vi "Clear Faults Test.vi"() -> ()   [LabVIEW 2014]
uses:
  Controls/Gen Data.ctl
  Controls/ES System Data.ctl
  Controls/StringSelector.ctl
  Controls/PC Data.ctl
  Controls/MicroZed Config Op Mode.ctl
  Controls/FPGA Data.ctl
panel:
  out "Startup":bool
  out "Wait for Fault":bool
  in  "Shutdown?":bool
  out "Error Out":errorcluster
  out "Clear Error":bool
  out "Manual Shutdown":bool
  in  "Error In":errorcluster
  in  "FPGA Data":T1 {"SSG Active Current" format="%2.1f"; "PV Reactive Power (L1)" format="%2.1f"; "PV Reactive Power (L2)" format="%2.1f"; "PV Total Reactive Power" format="%2.1f"; "Gen Reactive Power (L1)" format="%2.1f"; "Gen Reactive Power (L2)" format="%2.1f"; "Gen Total Reactive Power" format="%2.1f"; "SSG Reactive Power (L1)" format="%2.1f"; "SSG Reactive Power (L2)" format="%2.1f"; "SSG Total Reactive Power" format="%2.1f"; "PV Total Current" format="%2.1f"; "PV Total Voltage" format="%2.1f"; "PV Active Power (L1)" format="%2.1f"; "PV Active Power (L2)" format="%2.1f"; "PV App Power (L1)" format="%2.1f"; "PV App Power (L2)" format="%2.1f"; "PV Total Active Power" format="%2.1f"; "PV Total App Power" format="%2.1f"; "PV Arms (L1)" format="%2.1f"; "PV Arms (L2)" format="%2.1f"; "PV Vrms (L1)" format="%2.1f"; "PV Vrms (L2)" format="%2.1f"; "Gen Total Current" format="%2.1f"; "SSG Total Current" format="%2.1f"; "Gen Total Voltage" format="%2.1f"; "SSG Total Voltage" format="%2.1f"; "Gen Active Power (L1)" format="%2.1f"; "Gen Active Power (L2)" format="%2.1f"; "SSG Active Power (L1)" format="%2.1f"; "SSG Active Power (L2)" format="%2.1f"; "Gen App Power (L1)" format="%2.1f"; "Gen App Power (L2)" format="%2.1f"; "SSG App Power (L1)" format="%2.1f"; "SSG App Power (L2)" format="%2.1f"; "Gen Total Active Power" format="%2.1f"; "Gen Total App Power" format="%2.1f"; "Gen Arms (L1)" format="%2.1f"; "Gen Arms (L2)" format="%2.1f"; "Gen Vrms (L1)" format="%2.1f"; "Gen Vrms (L2)" format="%2.1f"; "SSG Total Active Power" format="%2.1f"; "SSG Total App Power" format="%2.1f"; "SSG Arms (L1)" format="%2.1f"; "SSG Arms (L2)" format="%2.1f"; "SSG Vrms (L1)" format="%2.1f"; "SSG Vrms (L2)" format="%2.1f"}
  in  "PC Data":T2 {"Alarms 2" format="%016b"; "Faults 2" format="%016b"; "Alarms 1" format="%016b"; "Faults 1" format="%016b"; "Contactor FB" format="%.0b"; "DC Voltage SP" format="%2.1f"; "Clear Faults SP" format="%.0b"; "Neutral Current" format="%2.1f"; "AC Current - L2" format="%2.1f"; "AC Voltage - L2" format="%2.1f"; "Temperature" format="%2.1f"; "DC Voltage" format="%2.1f"; "AC Current SP" format="%2.1f"; "AC Voltage SP" format="%2.1f"; "Frequency SP" format="%2.1f"; "AC Frequency" format="%2.1f"; "AC Current - L1" format="%2.1f"; "AC Voltage- L1" format="%2.1f"}
  in  "ES System Data":T4={"Voltage"=0.0, "Current"=0.0, "SOC Avg"=0.0, "Faults"=0, "Alarms"=0, "# Strings"=0, "Max Temp"=0, "Min Temp"=0, "Max Cell Voltage"=0.0, "Min Cell Voltage"=0.0, "Energy Capacity"=0.0, "Energy Remaining"=0.0, "SOC Min"=0.0, "SOC Max"=0.0, "ES Fault"=FALSE, "String Select"=enum."3 Strings", "ES Com Fault"=FALSE, "SOH Avg"=0.0}
  in  "Gen Active":T6 {"Alarms" format="%04x"}
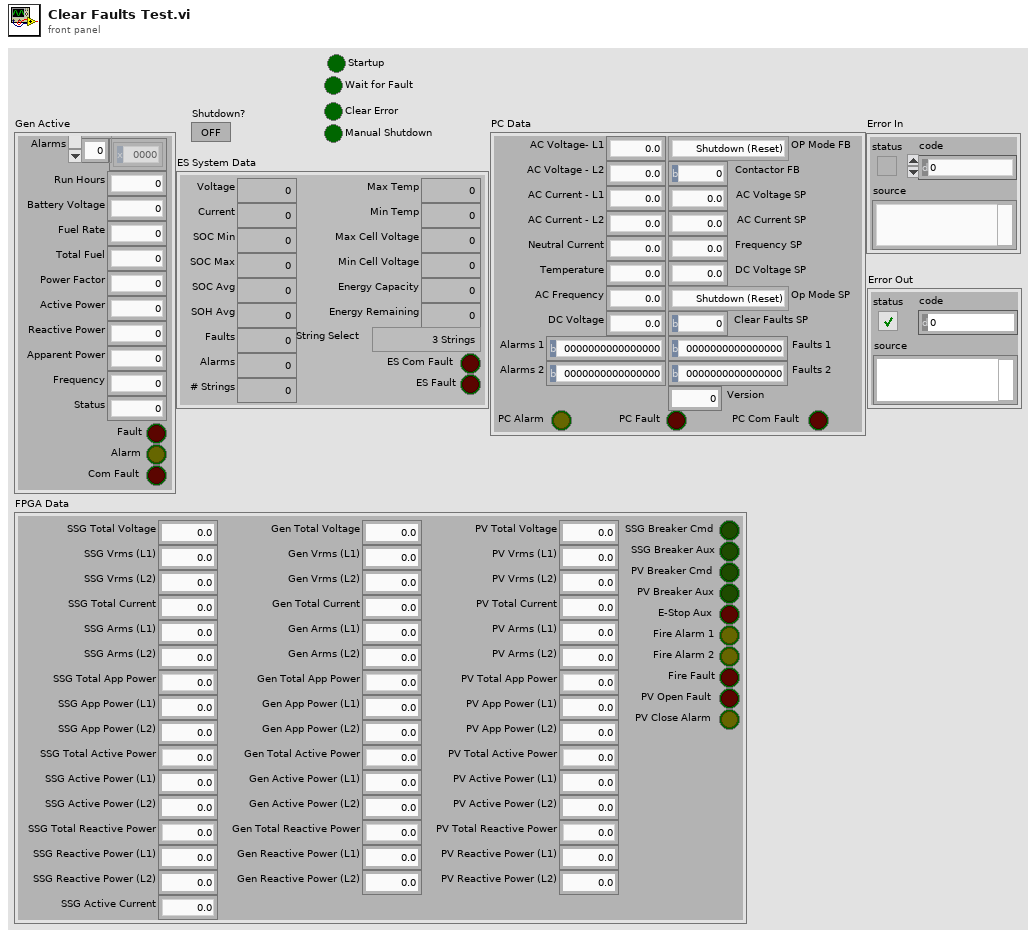
[diagram p1: front panel]
types:
  T1 = typedef "FPGA Data.ctl" = cluster{"Gen Total Voltage":dbl, "Gen Vrms (L1)":dbl, "Gen Vrms (L2)":dbl, "Gen Total Current":dbl, "Gen Arms (L1)":dbl, "Gen Arms (L2)":dbl, "Gen Total App Power":dbl, "Gen App Power (L1)":dbl, "Gen App Power (L2)":dbl, "Gen Total Active Power":dbl, "Gen Active Power (L1)":dbl, "Gen Active Power (L2)":dbl, "Gen Total Reactive Power":dbl, "Gen Reactive Power (L1)":dbl, "Gen Reactive Power (L2)":dbl, "SSG Total Voltage":dbl, "SSG Vrms (L1)":dbl, "SSG Vrms (L2)":dbl, "SSG Total Current":dbl, "SSG Arms (L1)":dbl, "SSG Arms (L2)":dbl, "SSG Total App Power":dbl, "SSG App Power (L1)":dbl, "SSG App Power (L2)":dbl, "SSG Total Active Power":dbl, "SSG Active Power (L1)":dbl, "SSG Active Power (L2)":dbl, "SSG Total Reactive Power":dbl, "SSG Reactive Power (L1)":dbl, "SSG Reactive Power (L2)":dbl, "PV Total Voltage":dbl, "PV Vrms (L1)":dbl, "PV Vrms (L2)":dbl, "PV Total Current":dbl, "PV Arms (L1)":dbl, "PV Arms (L2)":dbl, "PV Total App Power":dbl, "PV App Power (L1)":dbl, "PV App Power (L2)":dbl, "PV Total Active Power":dbl, "PV Active Power (L1)":dbl, "PV Active Power (L2)":dbl, "PV Total Reactive Power":dbl, "PV Reactive Power (L1)":dbl, "PV Reactive Power (L2)":dbl, "SSG Breaker Cmd":bool, "SSG Breaker Aux":bool, "PV Breaker Cmd":bool, "PV Breaker Aux":bool, "E-Stop Aux":bool, "Fire Alarm 1":bool, "Fire Alarm 2":bool, "Fire Fault":bool, "PV Open Fault":bool, "PV Close Alarm":bool, "SSG Active Current":dbl}
  T2 = typedef "PC Data.ctl" = cluster{"AC Voltage- L1":dbl, "AC Voltage - L2":dbl, "AC Current - L1":dbl, "AC Current - L2":dbl, "Neutral Current":dbl, "Temperature":dbl, "AC Frequency":dbl, "DC Voltage":dbl, "AC Voltage SP":dbl, "AC Current SP":dbl, "Frequency SP":dbl, "Op Mode SP":T3, "Clear Faults SP":u16, "PC Com Fault":bool, "PC Fault":bool, "DC Voltage SP":dbl, "OP Mode FB":T3, "Contactor FB":u16, "Faults 1":u16, "Alarms 1":u16, "Faults 2":u16, "Alarms 2":u16, "PC Alarm":bool, "Version":u16}
  T3 = typedef "MicroZed Config Op Mode.ctl" = enum16{"Shutdown (Reset)", "Startup", "Idle", "Voltage Mode", "Current Mode", "Fault", "OL Voltage (Debug)", "No Data"}
  T4 = typedef "ES System Data.ctl" = cluster{"Voltage":sgl, "Current":sgl, "SOC Avg":sgl, "Faults":u16, "Alarms":u16, "# Strings":u16, "Max Temp":i16, "Min Temp":i16, "Max Cell Voltage":sgl, "Min Cell Voltage":sgl, "Energy Capacity":sgl, "Energy Remaining":sgl, "SOC Min":sgl, "SOC Max":sgl, "ES Fault":bool, "String Select":T5, "ES Com Fault":bool, "SOH Avg":sgl}
  T5 = typedef "StringSelector.ctl" = enum16{"1 String (1)", "1 String (2)", "1 String (3)", "2 Strings (1 2)", "2 Strings (2 3)", "2 Strings (1 3)", "3 Strings"}
  T6 = typedef "Gen Data.ctl" = cluster{"Alarms":i16[], "Run Hours":dbl, "Battery Voltage":dbl, "Fuel Rate":dbl, "Total Fuel":dbl, "Power Factor":dbl, "Active Power":dbl, "Reactive Power":dbl, "Apparent Power":dbl, "Frequency":dbl, "Status":u16, "Fault":bool, "Alarm":bool, "Com Fault":bool}
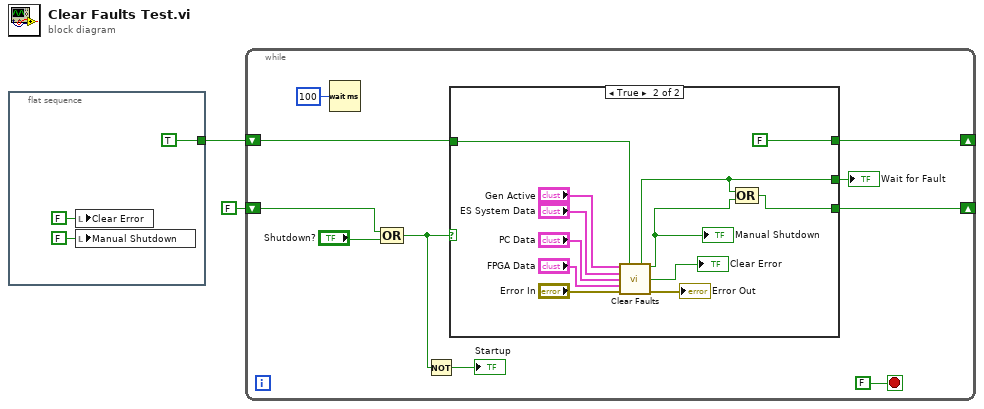
[diagram p0: block diagram]
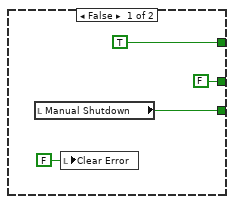
[diagram p2: hidden frame]
diagram:
  n1 = flat-sequence {
    tunnel: [TRUE] -> w2
    frame #0 {
      n2 = local write "Clear Error"(FALSE ("Clear Error")) -> ()
      n3 = local write "Manual Shutdown"(FALSE ("Manual Shutdown")) -> ()
    }
  }
  n4 = while {
    shift-right: [w12] -> _
    shift-left: w2 -> [w13]
    shift-right: [w11] -> _
    shift-left: FALSE ("Manual Shutdown") -> [w9]
    stop <- FALSE stop-if-true
    n5 = Wait (ms)(milliseconds to wait=u32 100) -> ()  [unwired: 1 out]
    n6 = Compound Arithmetic op=OR(w9, "Shutdown?") -> (w7:bool)
    n7 = Not(x=w7) -> (.not. x?=→"Startup":bool)
    n8 = case shown="True" w7 {
      tunnel: w13 -> [_ w24]
      tunnel: [TRUE FALSE] -> w12
      tunnel: [w18 w20] -> w11
      tunnel: [FALSE ("Wait for Fault") w22] -> w8
      frame False {
        n9 = local read "Manual Shutdown"() -> (w18:bool)
        n10 = local write "Clear Error"(FALSE ("Clear Error")) -> ()
      }
      frame True {
        n11 = call "Clear Faults.vi"("Gen Active"="Gen Active", "Initialize"=w24, "ES System Data"="ES System Data", "PC Data"="PC Data", "FPGA Data"="FPGA Data", "Error In"="Error In") -> ("Wait for Fault"=w22:bool, "Automatic Restart Fault"=w21:bool, "Clear Error"=→"Clear Error":bool, "Error Out"=→"Error Out":errorcluster)  [unwired: 6 in]
        "Manual Shutdown" <- w21
        n12 = Compound Arithmetic op=OR(w22, w21) -> (w20:bool)
      }
    }
    "Wait for Fault" <- w8
  }
